vi "MB Serial Example Master (Legacy).vi"() -> ()   [LabVIEW 2023, in "Voegtlin_NI_SMART_Modbus_Drivers.lvlib"]
uses:
  Voegtlin_NI_SMART_Modbus_Drivers.lvlib
  MB Modbus Command.ctl
panel:
  in  "Stop":bool
  out "Slave Input Registers":u16[](array[numeric]) caption="Slave Input Registers (Read Only)"
  out "Slave Discrete Inputs":bool[](array[boolean])
  in  "Coils to Write":bool[](array[boolean])=[FALSE, FALSE, FALSE, FALSE]
  in  "Registers to Write":u16[](array[numeric])=[0, 0, 0, 0]
  in  "VISA resource name":refnum<visa-resource-name>
  # "MB Serial Example Master.vi\n\nInstructions\n1. Connect your 2 COMs ports using a cross-over cable\n2. Select a COM port in VISA resouce name\n3. Open and run MB Example Slave.vi\n4. Run this VI.\n5. Modify the discrete inputs or input registers on the slave -> they're updated on the master.\n6. Modify the coils and registers on the master -> they're updated on the slave."
  # "Data to write to the slave"
  # "Slave Read-only Registers"
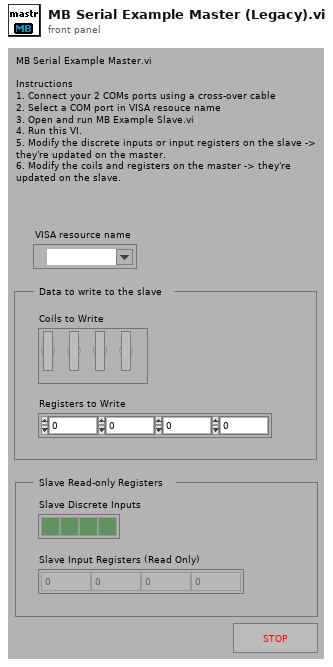
[diagram p1: front panel]
types:
  T1 = cluster{"Mode":enum16{"RTU", "ASCII"}, "Slave Address":u8}
  T2 = typedef "Voegtlin_NI_SMART_Modbus_Drivers.lvlib/MB Modbus Command.ctl" = cluster{"Function Code":u8, "Starting Address":u16, "Quantity":u16, "Data":u16[], "Discrete":bool[]}
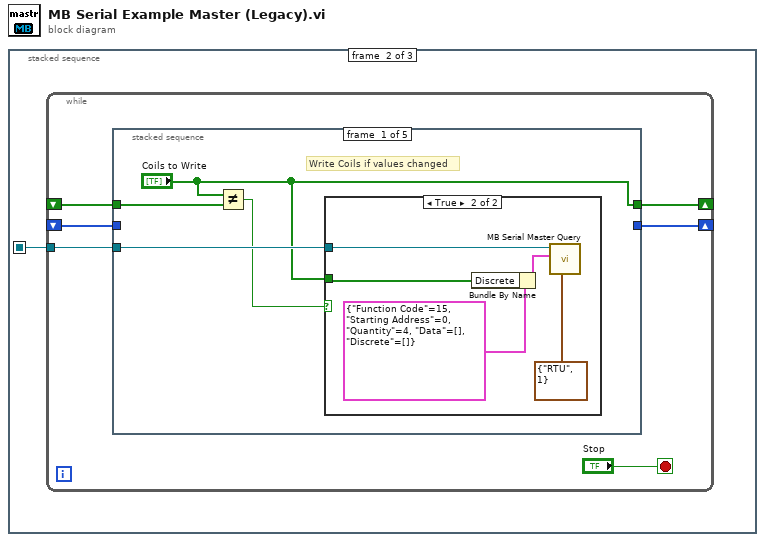
[diagram p0: block diagram]
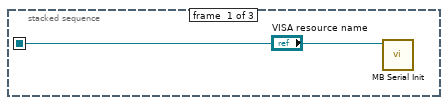
[diagram p2: hidden frame]
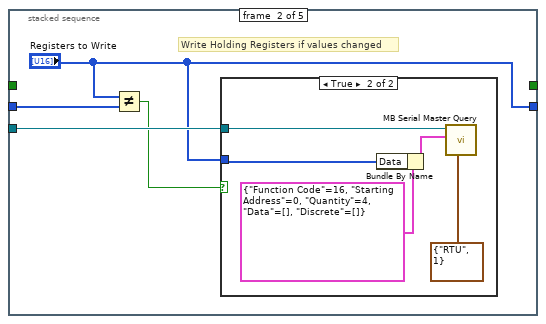
[diagram p4: hidden frame]
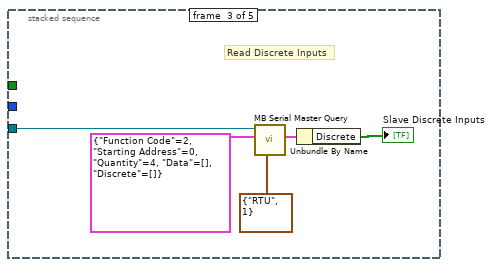
[diagram p6: hidden frame]
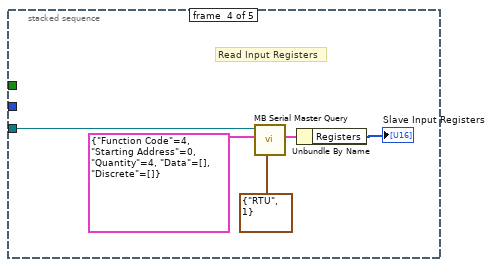
[diagram p7: hidden frame]
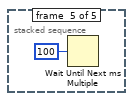
[diagram p8: hidden frame]
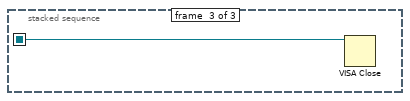
[diagram p9: hidden frame]
diagram:
  n1 = stacked-sequence {
    seq-local: ["VISA resource name" _ _] -> [_ w2 w38]
    frame #0 {
      n2 = call "MB Serial Init.vi"("VISA resource name"="VISA resource name") -> ()  [unwired: 6 in, 5 out]
    }
    frame #1 {
      n3 = while {
        tunnel: w2 -> [w8]
        shift-right: [w6] -> _
        shift-left: _ -> [w7]
        shift-right: [w4] -> _
        shift-left: _ -> [w5]
        stop <- "Stop" stop-if-true
        n4 = stacked-sequence {
          tunnel: w8 -> [w12 w21 w31 w36 _]
          tunnel: w7 -> [w11 _ _ _ _]
          tunnel: ["Coils to Write" _ _ _ _] -> w6
          tunnel: w5 -> [_ w19 _ _ _]
          tunnel: [_ "Registers to Write" _ _ _] -> w4
          frame #0 {
            # "Write Coils if values changed"
            n5 = Not Equal?(x="Coils to Write", y=w11) -> (x != y?=w9:bool)
            n6 = case shown="True" w9 {
              tunnel: w12 -> [_ w14]
              tunnel: "Coils to Write" -> [_ w13]
              frame False {
              }
              frame True {
                n7 = Bundle By Name(cluster=T2 {"Function Code"=15, "Starting Address"=0, "Quantity"=4, "Data"=[], "Discrete"=[]} ("MODBUS Command"), "Discrete"=w13) -> (w16:T2)
                n8 = call "MB Serial Master Query.vi"("Serial Parameters"=T1 {"Mode"=enum."RTU", "Slave Address"=1}, "Modbus Command"=w16, "VISA resource name"=w14) -> ()  [unwired: 4 in, 5 out]
              }
            }
          }
          frame #1 {
            # "Write Holding Registers if values changed"
            n9 = Not Equal?(x="Registers to Write", y=w19) -> (x != y?=w20:bool)
            n10 = case shown="True" w20 {
              tunnel: w21 -> [_ w23]
              tunnel: "Registers to Write" -> [_ w22]
              frame False {
              }
              frame True {
                n11 = Bundle By Name(cluster=T2 {"Function Code"=16, "Starting Address"=0, "Quantity"=4, "Data"=[], "Discrete"=[]} ("MODBUS Command"), "Data"=w22) -> (w25:T2)
                n12 = call "MB Serial Master Query.vi"("Serial Parameters"=T1 {"Mode"=enum."RTU", "Slave Address"=1}, "Modbus Command"=w25, "VISA resource name"=w23) -> ()  [unwired: 4 in, 5 out]
              }
            }
          }
          frame #2 {
            # "Read Discrete Inputs"
            n13 = call "MB Serial Master Query.vi"("Serial Parameters"=T1 {"Mode"=enum."RTU", "Slave Address"=1}, "Modbus Command"=T2 {"Function Code"=2, "Starting Address"=0, "Quantity"=4, "Data"=[], "Discrete"=[]} ("MODBUS Command"), "VISA resource name"=w31) -> ("Registers"=w30:cluster{"Registers":u16[], "Discrete":bool[]})  [unwired: 4 in, 4 out]
            n14 = Unbundle By Name(w30) -> ("Discrete"=→"Slave Discrete Inputs":bool[])
          }
          frame #3 {
            # "Read Input Registers"
            n15 = call "MB Serial Master Query.vi"("Serial Parameters"=T1 {"Mode"=enum."RTU", "Slave Address"=1}, "Modbus Command"=T2 {"Function Code"=4, "Starting Address"=0, "Quantity"=4, "Data"=[], "Discrete"=[]} ("MODBUS Command"), "VISA resource name"=w36) -> ("Registers"=w35:cluster{"Registers":u16[], "Discrete":bool[]})  [unwired: 4 in, 4 out]
            n16 = Unbundle By Name(w35) -> ("Registers"=→"Slave Input Registers":u16[])
          }
          frame #4 {
            n17 = Wait Until Next ms Multiple(millisecond multiple=u32 100) -> ()  [unwired: 1 out]
          }
        }
      }
    }
    frame #2 {
      n18 = VISA Close(VISA resource name=w38) -> ()  [unwired: 1 in, 1 out]
    }
  }
